vi "act-0026-01.vi"   [LabVIEW 2010]
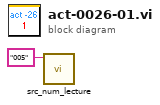
[diagram p0: block diagram]
diagram:
  n1 = call "src_num_lecture.vi"("src"="005") -> ()  [unwired: 6 in, 5 out]
